vi "setWifiSSID.vi"(8 "error":errorcluster, 10 "SSID":string, 11 "connection ID":refnum<k5>) -> (0 "error out":errorcluster, 3 "connection ID out":refnum<k5>)   [LabVIEW 2016, in "amc_api.lvlib"]
doc: "Changes the SSID of the network hosted (mode: access point) or connected to (mode: client)."
uses:
  amc_api.lvlib
panel:
  out "jsonRespIn":string
  out "JSON-response":string="{\"jsonrpc\":\"2.0\",\"method\":\"\",\"params\":[5,1.245,true,\"name\"],\"id\":\"1\"}"
  out "JSON request":string
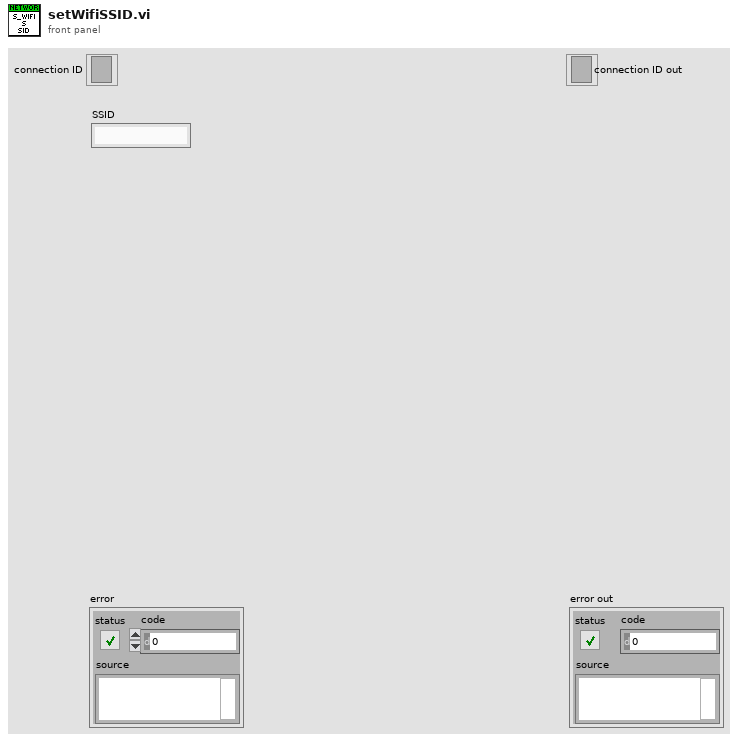
[diagram p1: front panel]
types:
  T1 = cluster{"jsonrpc":string, "method":string, "params":string[], "id":string, "api":i32, "pid":string}
  T2 = enum16{"Standard", "Buffered", "CRLF", "Immediate"}
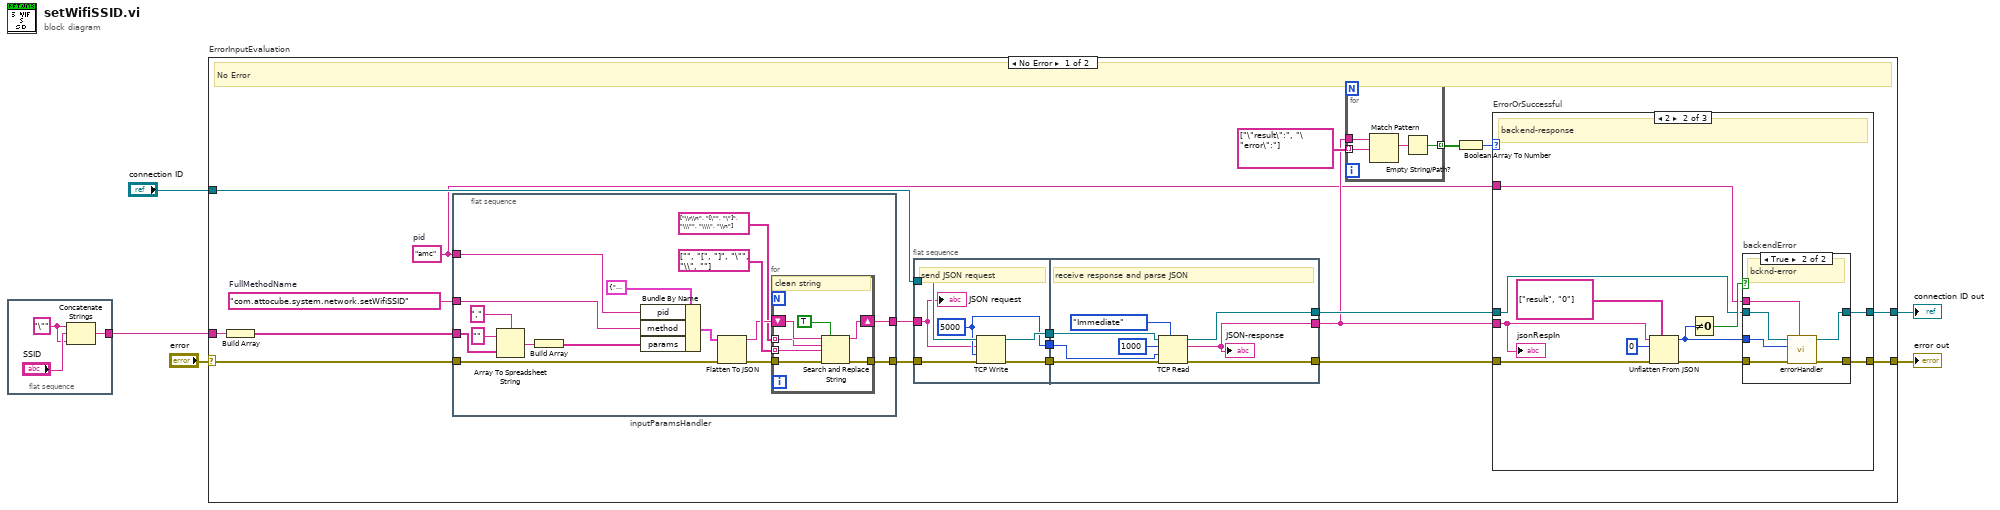
[diagram p0: block diagram]
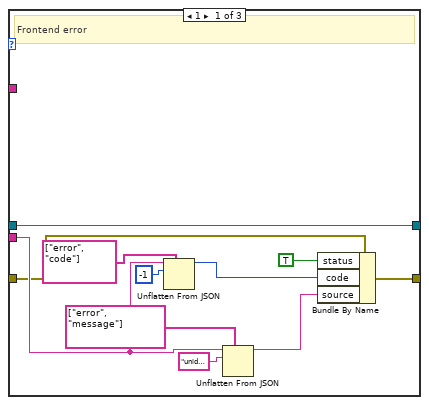
[diagram p2: hidden frame]
diagram:
  n1 = flat-sequence "in_string" {
    tunnel: [w7] -> w1
    frame #0 {
      w6 = "\"" ("string")
      n2 = Concatenate Strings(w6, "SSID", w6) -> (w7:string)
    }
  }
  n3 = case "ErrorInputEvaluation" shown="No Error" "error" {
    selector: "error" -> [w14 w101]
    tunnel: "connection ID" -> [w24 w102]
    tunnel: [w16 w101] -> w4
    tunnel: [w17 w102] -> w3
    tunnel: w1 -> [w9 _]
    frame No Error {
      w10 = "amc"  # pid
      w15 = "com.attocube.system.network.setWifiSSID"  # FullMethodName
      # "No Error"
      n4 = Build Array ("ParametersArrayString")(w9) -> (w13:string[])
      n5 = flat-sequence "inputParamsHandler" {
        tunnel: [w33] -> w12
        tunnel: w13 -> [w39]
        tunnel: w14 -> [w38]
        tunnel: [w35] -> w11
        tunnel: w15 -> [w29]
        tunnel: w10 -> [w28]
        frame #0 {
          n6 = Array To Spreadsheet String(delimiter (Tab)=",", array=w39, 3:"" ("format string")) -> (spreadsheet string=w41:string)
          n7 = Build Array "Build Array"(w41) -> (w30:string[])
          n8 = Bundle By Name(cluster=T1 {"jsonrpc"="2.0", "method"="com.attocube.amc.res.setRESReadOutFreq", "params"=[], "id"="1", "api"=2, "pid"=""}, "pid"=w28, "method"=w29, "params"=w30) -> (w40:T1)
          n9 = Flatten To JSON(anything=w40, error in (no error)=w38) -> (JSON string=w34:string, 11:w36:errorcluster)  [unwired: 1 in]
          n10 = for {
            tunnel: string[] ["\\r\\n", "[\"", "\"]", "\\\"", "\\\\", "\\n"] ("search string") -> [w47] mode=indexing
            tunnel: string[] ["", "[", "]", "\"", "\\", ""] ("replace string (\"\")") -> [w46] mode=indexing
            shift-right: [w49] -> w33
            shift-left: w34 -> [w48]
            tunnel: w36 -> [w45]
            tunnel: [w44] -> w35
            # "clean string"
            n11 = Search and Replace String(replace all?=TRUE ("replace all? (F)"), input string=w48, search string=w47, replace string=w46, error in=w45) -> (result string=w49:string, error out=w44:errorcluster)  [unwired: 3 in, 2 out]
          }
        }
      }
      n12 = flat-sequence {
        tunnel: w24 -> [w92]
        tunnel: [w90] -> w27
        tunnel: [w91] -> w26
        tunnel: w11 -> [w87]
        tunnel: [w89] -> w25
        tunnel: w12 -> [w88]
        tunnel: [w96] -> w20
        tunnel: w27 -> [w98]
        tunnel: w26 -> [w97]
        tunnel: [w94] -> w19
        tunnel: w25 -> [w95]
        tunnel: [w93] -> w18
        frame #0 {
          w89 = 5000 ("timeout ms (25000)")
          # "send JSON request"
          n13 = TCP Write(connection ID=w92, data in=w88, error in (no error)=w87, 9:w89) -> (connection ID out=w90:refnum<k5>, error out=w91:errorcluster)  [unwired: 1 out]
          "JSON request" <- w88
        }
        frame #1 {
          # "receive response and parse JSON"
          n14 = TCP Read(connection ID=w98, bytes to read=1000, error in (no error)=w97, 7:T2."Immediate" ("mode (standard)"), 9:w95) -> (connection ID out=w96:refnum<k5>, data out=w93:string, error out=w94:errorcluster)
          "JSON-response" <- w93
        }
      }
      n15 = for {
        tunnel: string[] ["\"result\":", "\"error\":"] ("path") -> [w53] mode=indexing
        tunnel: [w51] -> w22 mode=indexing
        tunnel: w18 -> [w54]
        n16 = Match Pattern(string=w54, regular expression=w53) -> (match substring=w52:string)  [unwired: 1 in, 3 out]
        n17 = Empty String/Path?(string/path=w52) -> (empty?=w51:bool)
      }
      n18 = Boolean Array To Number(Boolean array=w22) -> (number=w21:u32)
      n19 = case "ErrorOrSuccessful" shown="2" w21 {
        tunnel: w18 -> [w57 w67 _]
        tunnel: w20 -> [w55 w70 w86]
        tunnel: [w55 w69 w86] -> w17
        tunnel: [w58 w68 w85] -> w16
        tunnel: w19 -> [w56 w71 w85]
        tunnel: w10 -> [_ w66 _]
        frame 1 {
          # "Frontend error"
          n20 = Unflatten From JSON(path=string[] ["error", "code"], JSON string=w57, type and defaults=-1) -> (value=w64:i32)  [unwired: 4 in, 1 out]
          n21 = Unflatten From JSON(path=string[] ["error", "message"], JSON string=w57, type and defaults="unidentified error") -> (value=w65:string)  [unwired: 4 in, 1 out]
          n22 = Bundle By Name(cluster=w56, "status"=TRUE, "code"=w64, "source"=w65) -> (w58:errorcluster)
        }
        frame 2 {
          # "backend-response"
          n23 = Unflatten From JSON(path=string[] ["result", "0"], JSON string=w67, type and defaults=0, error in (no error)=w71) -> (value=w76:i32, error out=w74:errorcluster)  [unwired: 3 in]
          n24 = Not Equal To 0?(x=w76) -> (x != 0?=w75:bool)
          n25 = case "backendError" shown="True" w75 {
            tunnel: w76 -> [_ w84]
            tunnel: w74 -> [w78 w83]
            tunnel: [w77 w82] -> w69
            tunnel: [w78 w81] -> w68
            tunnel: w70 -> [w77 w80]
            tunnel: w66 -> [_ w79]
            frame False {
              # "successful"
            }
            frame True {
              # "bcknd-error"
              n26 = call "errorHandler.vi"("pid"=w79, "error in"=w83, "errNbr"=w84, "connection ID"=w80) -> ("error out 2"=w81:errorcluster, "connection ID out"=w82:refnum<k5>)  [unwired: 6 in]
            }
          }
          "jsonRespIn" <- w67
        }
        frame Default {
          # "NoResponse"
        }
      }
    }
    frame Error {
      # "Error"
    }
  }
  "error out" <- w4
  "connection ID out" <- w3
